vi "DeInit.vi"(9 "GlobalDataRef":refnum<data-value>, 10 "Queues":T1) -> ()   [LabVIEW 2015]
uses:
  Telegram/Methods/TypeDefs/Message.ctl
  TypeDefs/GlobalData.ctl
  Telegram/Methods/TypeDefs/ReplyKeyboardMarkup.ctl
  <vilib>/FPGAPlugInAG/Dynamic/niLvFpga_Close_Dynamic.vi
  <vilib>/rvi/interface/nirviCloseFPGA/nirviCloseFPGA.xnode
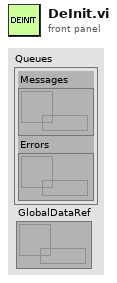
[diagram p1: front panel]
types:
  T1 = cluster{"Messages":refnum<queue>, "Errors":refnum<queue>}
  T2 = typedef "GlobalData.ctl" = cluster{"FPGA VI Ref":refnum<k20>, "Token":string, "ActiveChats":cluster{"ChatId":i32, "Type":string}[], "ActiveKeyboards":cluster{"Chat#":i32, "ReplyKeyboardMarkup":T3}[], "RefStringIn":refnum<vi>}
  T3 = typedef "ReplyKeyboardMarkup.ctl" = cluster{"keyboard":cluster{"text":string, "req_loc":bool}[][], "resize_keyboard":bool, "one_time_keyboard":bool, "selective":bool}
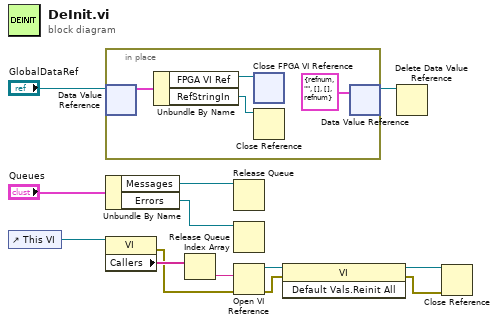
[diagram p0: block diagram]
diagram:
  n1 = control-ref of="This VI"() -> (w8:refnum<vi>)
  n2 = in-place {
    n3 = in-place-dvr #1("GlobalDataRef") -> (w17:T2)  [unwired: 1 out]
    n4 = Unbundle By Name(w17) -> ("FPGA VI Ref"=w16:refnum<k20>, "RefStringIn"=w15:refnum<vi>)
    n5 = xnode "Close FPGA VI Reference"("FPGA VI Reference In"=w16) -> ()  [unwired: 1 in, 1 out]
    n6 = Close Reference(reference=w15) -> ()  [unwired: 1 in, 1 out]
    n7 = in-place-dvr #1(T2 {"FPGA VI Ref"=refnum, "Token"="", "ActiveChats"=[], "ActiveKeyboards"=[], "RefStringIn"=refnum} ("data value")) -> (w12:refnum<data-value>)  [unwired: 1 out]
  }
  n8 = Unbundle By Name("Queues") -> ("Messages"=w10:refnum<queue>, "Errors"=w9:refnum<queue>)
  n9 = property class="VI"(reference=w8) -> (error out=w1:errorcluster, "Callers"=w7:string[])  [unwired: 1 in, 1 out]
  n10 = Index Array(array=w7) -> (element=w6:string)  [unwired: 1 in]
  n11 = Release Queue(queue=w10) -> ()  [unwired: 2 in, 3 out]
  n12 = Release Queue(queue=w9) -> ()  [unwired: 2 in, 3 out]
  n13 = Open VI Reference(vi path=w6, error in (no error)=w1) -> (vi reference=w5:refnum<vi>, error out=w3:errorcluster)  [unwired: 4 in]
  n14 = invoke class="VI" method="Default Vals.Reinit All"(reference=w5, error in=w3) -> (reference out=w4:refnum<vi>, error out=w2:errorcluster)  [unwired: 1 in, 1 out]
  n15 = Delete Data Value Reference(data value reference=w12) -> ()  [unwired: 1 in, 2 out]
  n16 = Close Reference(reference=w4, error in (no error)=w2) -> ()  [unwired: 1 out]
